vi "Preset distend cortices.vi"(11 "Vertex data":T1) -> (3 "Vertex data distended":T1)   [LabVIEW 2015, in "Morph Cortical Surfaces.lvlib"]
doc: "Preset distension settings to minimize horizon when viewing from lateral or medial side."
uses:
  Morph Cortical Surfaces.lvlib
  Vertex data control.ctl
  Distend mode.ctl
  Distend method control.ctl
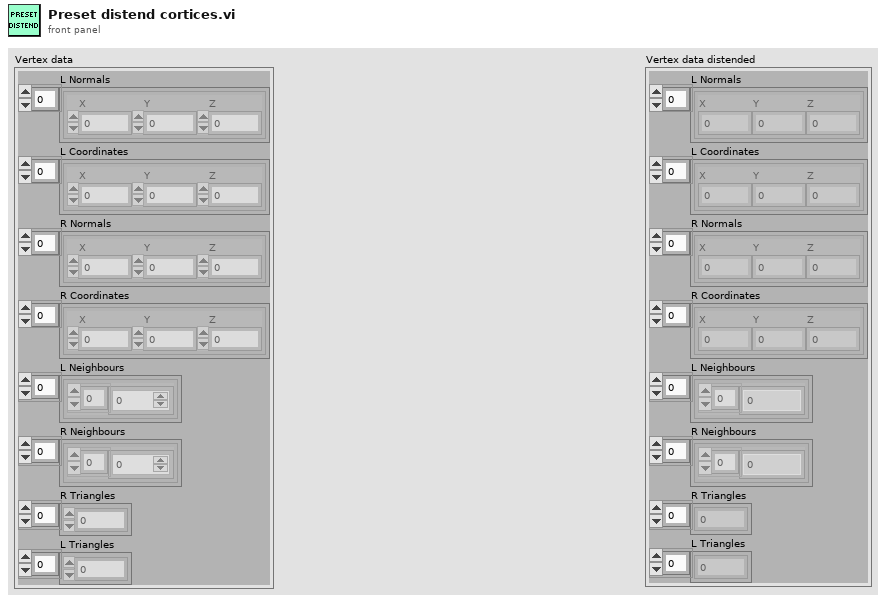
[diagram p1: front panel]
types:
  T1 = typedef "Morph Cortical Surfaces.lvlib/Vertex data control.ctl" = cluster{"L Normals":cluster{"X":sgl, "Y":sgl, "Z":sgl}[], "L Coordinates":cluster{"X":sgl, "Y":sgl, "Z":sgl}[], "R Normals":cluster{"X":sgl, "Y":sgl, "Z":sgl}[], "R Coordinates":cluster{"X":sgl, "Y":sgl, "Z":sgl}[], "L Neighbours":cluster{i32[]}[], "R Neighbours":cluster{i32[]}[], "R Triangles":i32[], "L Triangles":i32[]}
  T2 = typedef "Morph Cortical Surfaces.lvlib/Distend mode.ctl" = enum16{"Morph Width", "Balloon Width", "Morph Height", "Balloon Height"}
  T3 = typedef "Morph Cortical Surfaces.lvlib/Distend method control.ctl" = enum16{"Use weighting values", "Linear distance from center", "Exponential distance from center"}
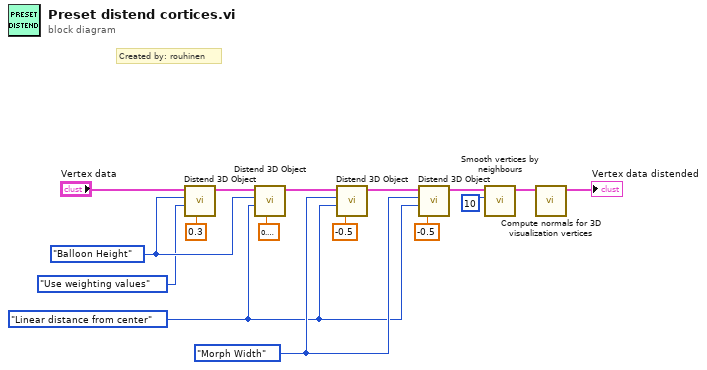
[diagram p0: block diagram]
diagram:
  w2 = Distend_mode."Morph Width" ("Distend mode")
  w1 = Distend_method_control."Linear distance from center" ("Distend method")
  w8 = Distend_mode."Balloon Height" ("Distend mode")
  # "Created by: rouhinen"
  n1 = call "Distend 3D Object.vi"("Distend size"=0.3, "Distend method"=Distend_method_control."Use weighting values", "Distend mode"=w8, "Normals and Coordinates"="Vertex data") -> ("Normals and Coordinates out"=w14:T1)  [unwired: 7 in]
  n2 = call "Distend 3D Object.vi"("Distend size"=0.19999999999999998, "Distend method"=w1, "Distend mode"=w8, "Normals and Coordinates"=w14) -> ("Normals and Coordinates out"=w13:T1)  [unwired: 7 in]
  n3 = call "Distend 3D Object.vi"("Distend size"=-0.5, "Distend method"=w1, "Distend mode"=w2, "Normals and Coordinates"=w13) -> ("Normals and Coordinates out"=w12:T1)  [unwired: 7 in]
  n4 = call "Distend 3D Object.vi"("Distend size"=-0.5, "Distend method"=w1, "Distend mode"=w2, "Normals and Coordinates"=w12) -> ("Normals and Coordinates out"=w11:T1)  [unwired: 7 in]
  n5 = call "Smooth vertices by neighbours.vi"("Smoothing rounds"=10, "Vertex data"=w11) -> ("Vertex data smoothened"=w10:T1)  [unwired: 9 in]
  n6 = call "Compute normals for 3D visualization vertices.vi"("Vertex data"=w10) -> ("Vertex data new normals"=→"Vertex data distended":T1)  [unwired: 10 in]
